vi "Set Sleep Mode.vi"(8 "error in (no error)":errorcluster, 10 "Sleep?":bool, 11 "PWM in":refnum<class "LINX-PCA9685 PWM.lvclass">) -> (0 "error out":errorcluster, 3 "PWM out":refnum<class "LINX-PCA9685 PWM.lvclass">)   [LabVIEW 2020, in "LINX-PCA9685 PWM.lvclass"]
uses:
  LINX-PCA9685 PWM.lvclass
  LINX I2C/LINX I2C.lvclass
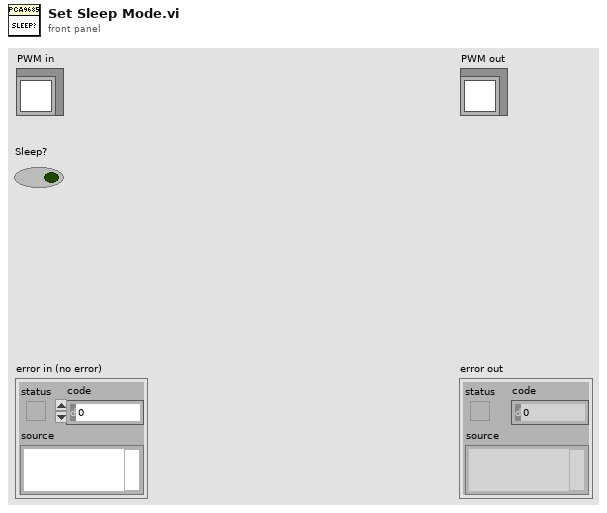
[diagram p1: front panel]
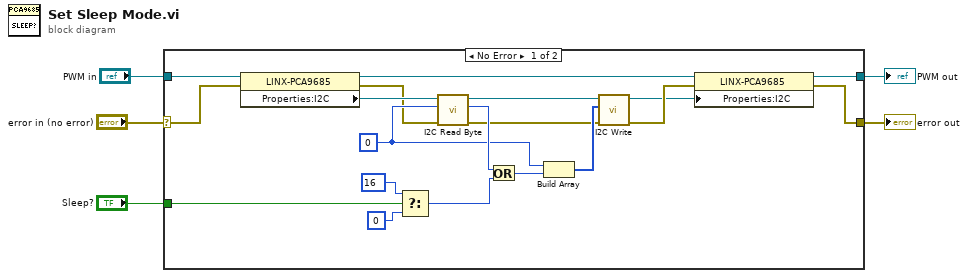
[diagram p0: block diagram]
diagram:
  n1 = case shown="No Error" "error in (no error)" {
    selector: "error in (no error)" -> [w11 w26]
    tunnel: [w7 w26] -> w4
    tunnel: [w10 w25] -> w2
    tunnel: "PWM in" -> [w13 w25]
    tunnel: "Sleep?" -> [w18 _]
    frame No Error {
      w20 = u8 0 ("Address")
      n2 = property class="LINX-PCA9685"(reference=w13, error in=w11) -> (reference out=w14:refnum<class "LINX-PCA9685 PWM.lvclass">, error out=w6:errorcluster, "Properties:I2C"=w12:refnum<class "LINX I2C.lvclass">)
      n3 = Select(t=u8 16 ("Address"), s=w18, f=u8 0 ("Address")) -> (s? t:f=w15:u8)
      n4 = call-dynamic "I2C Read Byte.vi"("error in (no error)"=w6, 10:w20, "LINX I2C in"=w12) -> ("error out"=w19:errorcluster, "Byte Read"=w23:u8, "LINX I2C out"=w24:refnum<class "LINX I2C.lvclass">)  [unwired: 6 in]
      n5 = Or(x=w23, y=w15) -> (x .or. y?=w22:u8)
      n6 = Build Array(w20, w22) -> (w21:u8[])
      n7 = call "I2C Write.vi"("error in (no error)"=w19, "Bytes to Write"=w21, "LINX I2C in"=w24) -> ("error out"=w9:errorcluster, "LINX I2C out"=w8:refnum<class "LINX I2C.lvclass">)  [unwired: 7 in]
      n8 = property class="LINX-PCA9685"(reference=w14, error in=w9, "Properties:I2C"=w8) -> (reference out=w10:refnum<class "LINX-PCA9685 PWM.lvclass">, error out=w7:errorcluster)
    }
    frame Error {
    }
  }
  "error out" <- w4
  "PWM out" <- w2
